vi "Launcher.vi"(8 "Quicklaunch (2)":bool, 9 "Launch Button (3)":bool, 10 "Launch Motors On (1)":bool) -> ()   [LabVIEW 2012]
uses:
  <vilib>/Rock Robotics/WPI/Solenoid/WPI_SolenoidValue.ctl
  <vilib>/Rock Robotics/WPI/Relay/WPI_RelayValue.ctl
  <vilib>/Rock Robotics/WPI/Solenoid/WPI_SolenoidSetEnum.vi
panel:
  out "Launcher On?":bool
  out "Launch Reduction":dbl
  in  "On Button Clicks":dbl
  out "Charge Up tick":dbl
  in  "Quicklaunch State":T1(ring)
  in  "Fast-Slow Variable":dbl=1.0
  in  "Charge Up Time":dbl=4000.0
  in  "Time Between Launches":dbl=2500.0
  out "Time Between tick":dbl
  out "Launch Wait tick":dbl
  in  "Launch Wait Time":dbl=500.0
  out "tick 2":dbl
  in  "time extended":dbl=500.0
  out "tick":dbl
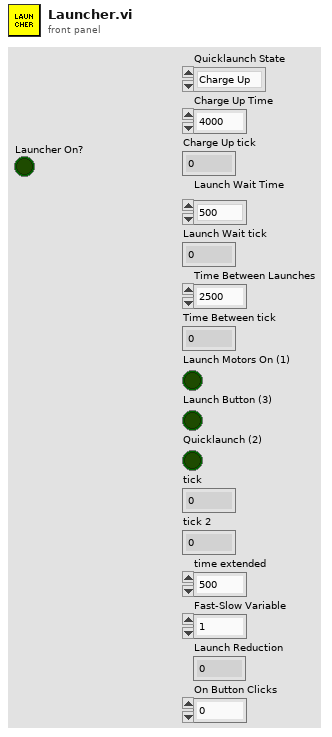
[diagram p1: front panel]
types:
  T1 = enum16{"Charge Up ", "Fire 1", "wait1", "Fire 2", "wait2", "Fire 3", "wait3", "Fire 4"}
  T2 = typedef "WPI_SolenoidValue.ctl" = enum16{"Off", "On", "Forward", "Reverse"}
  T3 = typedef "WPI_SolenoidDevRef.ctl" = cluster{"DevStatus":errorcluster, "Solenoid Module":T4, "Forward Solenoid Channel":T5, "Reverse Solenoid Channel":T5}
  T4 = typedef "FPGA_TypedefSolenoidModule.ctl" = enum16{"Solenoid Module 1", "Solenoid Module 2"}
  T5 = typedef "WPI_SolenoidChannel.ctl" = enum8{"Solenoid 1", "Solenoid 2", "Solenoid 3", "Solenoid 4", "Solenoid 5", "Solenoid 6", "Solenoid 7", "Solenoid 8", "Invalid"}
  T6 = typedef "WPI_RelayValue.ctl" = enum16{"Off", "On", "Forward", "Reverse"}
  T7 = typedef "WPI_MotorControlDeviceRef.ctl" = cluster{"DeviceStatus":errorcluster, "Type":enum16{"PWM", "CAN"}, "PWM":cluster{"Digital Module":T8, "PWM Channel":T9, "DeadBand":T10}, "CAN":cluster{"Device Number":u8, "Control Mode":T11, "Semaphore":T12, "Max Vout":dbl}, "Invert":bool, "TransformRef":T13, "InvTransformRef":T13}
  T8 = typedef "FPGA_TypedefDigitalModule.ctl" = enum16{"Digital Module 1", "Digital Module 2"}
  T9 = typedef "FPGA_DIOPWMChannel.ctl" = enum8{"PWM 1", "PWM 2", "PWM 3", "PWM 4", "PWM 5", "PWM 6", "PWM 7", "PWM 8", "PWM 9", "PWM 10", "Invalid"}
  T10 = typedef "WPI_PWMDeadband.ctl" = cluster{"Name":string, "maxPositivePwm":i32, "minPositivePwm":i32, "centerPwm":i32, "maxNegativePwm":i32, "minNegativePwm":i32, "angularRange":u16}
  T11 = typedef "WPI_CANJaguar_ControlMode.ctl" = enum8{"Percent VBus", "Current", "Speed", "Position", "Voltage"}
  T12 = typedef "Semaphore RefNum" = refnum<k1>
  T13 = typedef "WPI_PWMTransform_ConPane.ctl" = refnum<vi>
  T14 = typedef "WPI_RelayDevRef.ctl" = cluster{"DevStatus":errorcluster, "Relay Channel":T15, "Digital Module":T8, "Relay Direction":T16}
  T15 = typedef "FPGA_DIORelayChannel.ctl" = enum8{"Relay 1", "Relay 2", "Relay 3", "Relay 4", "Relay 5", "Relay 6", "Relay 7", "Relay 8", "Invalid"}
  T16 = typedef "WPI_RelayDirection.ctl" = enum16{"Both directions", "Forward only", "Reverse only"}
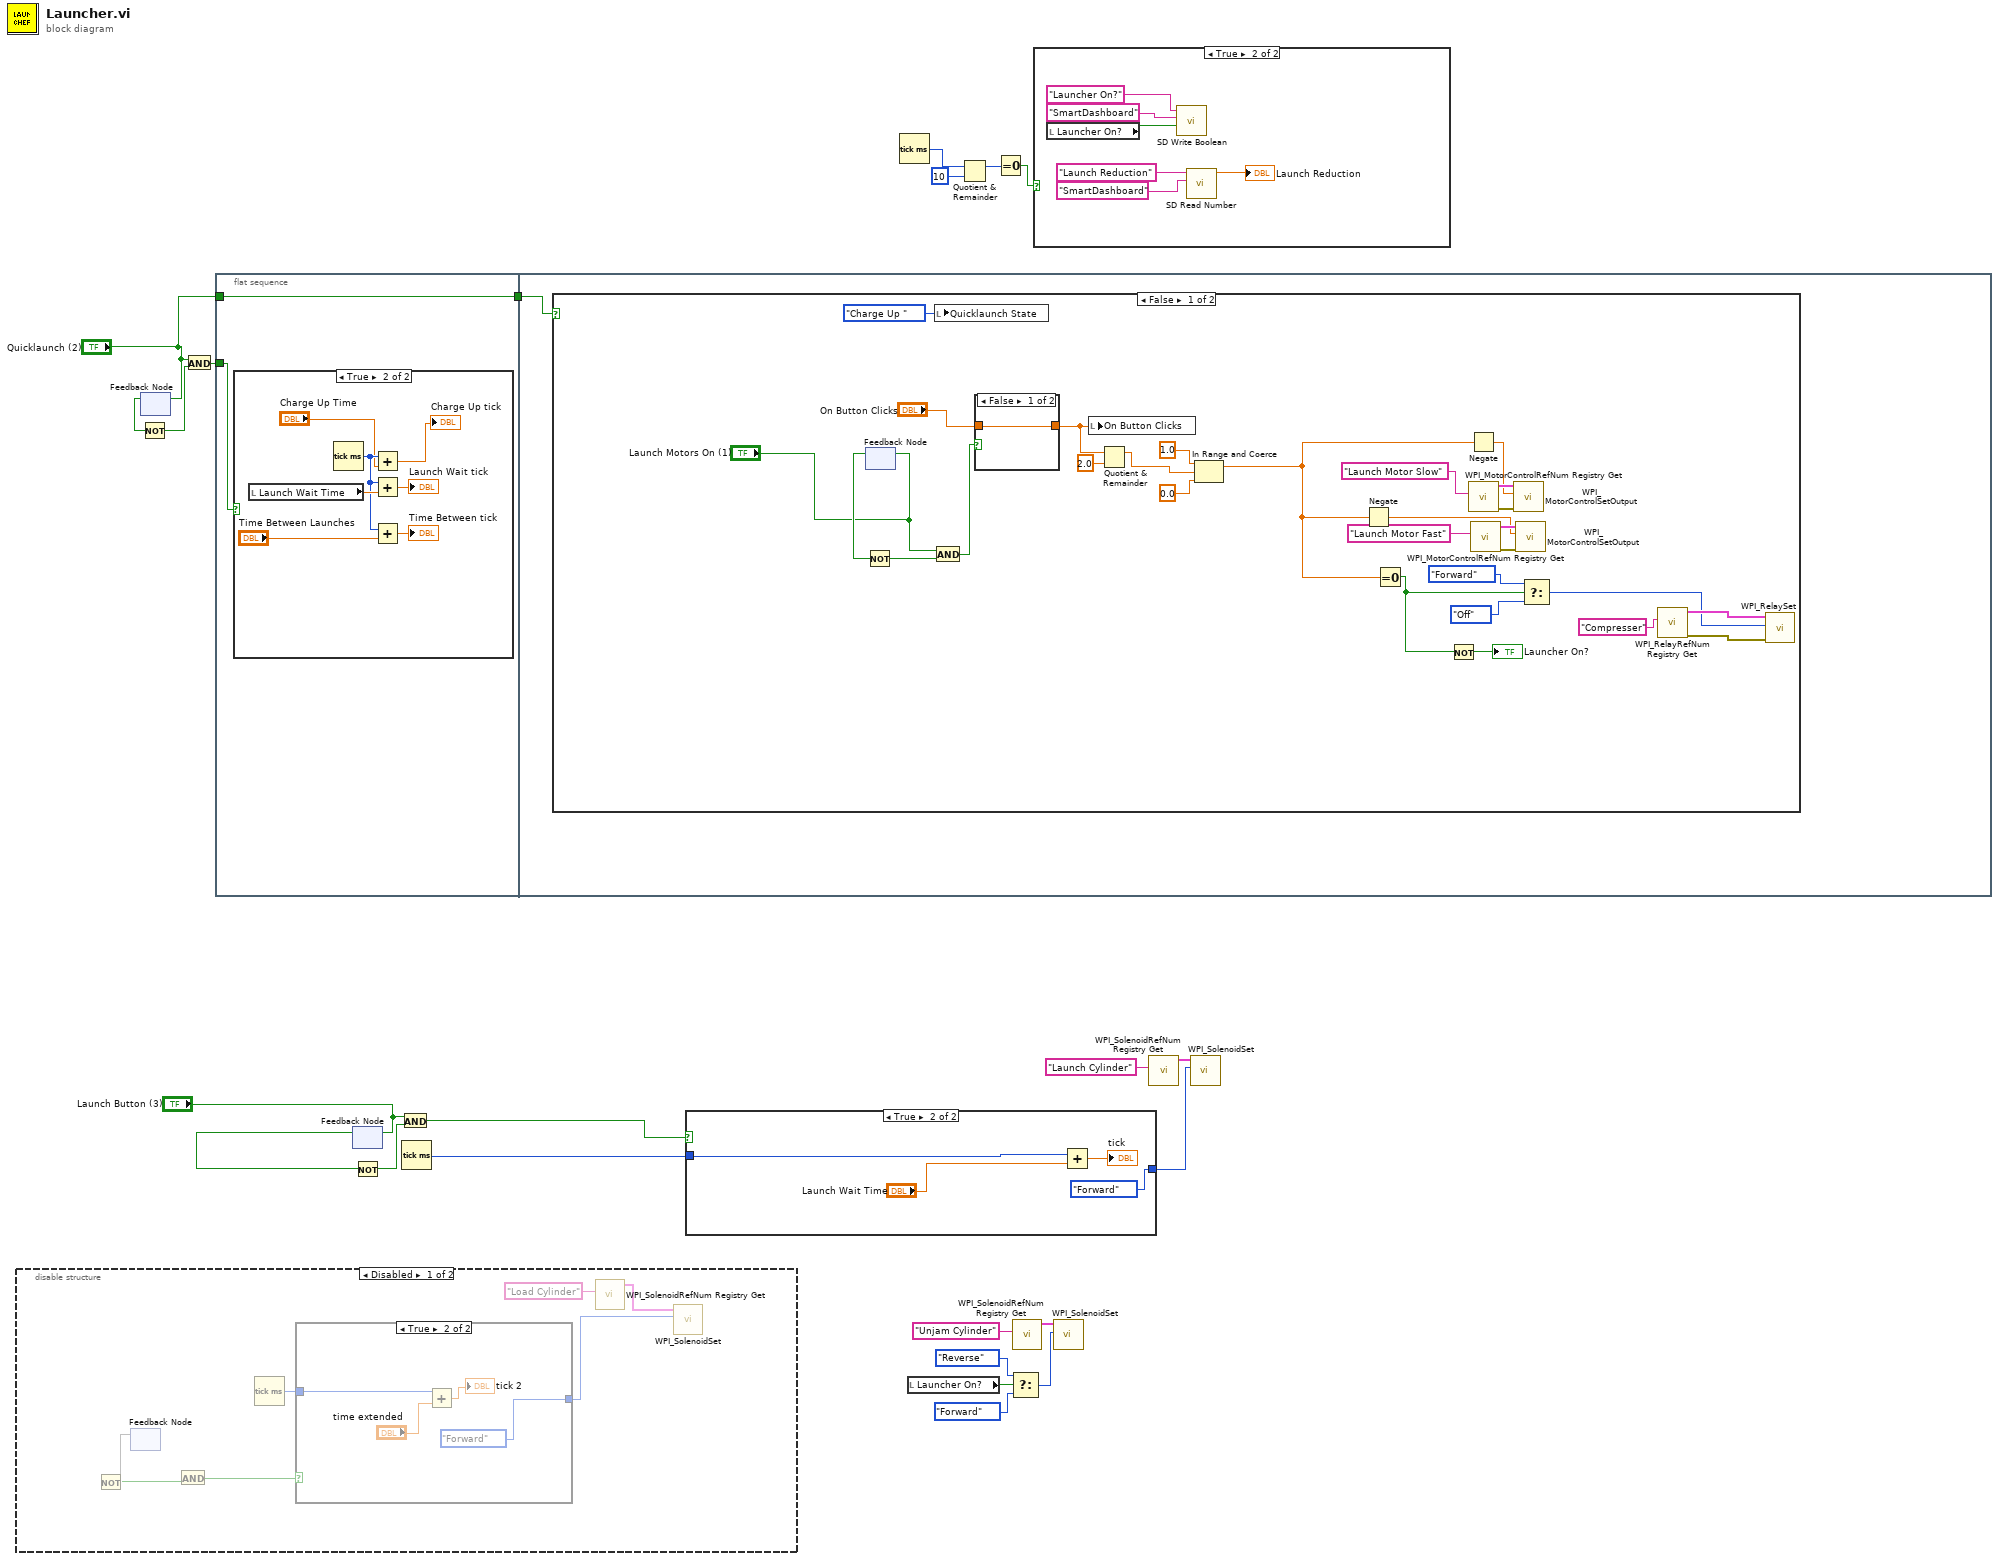
[diagram p0: block diagram]
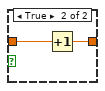
[diagram p4: hidden frame]
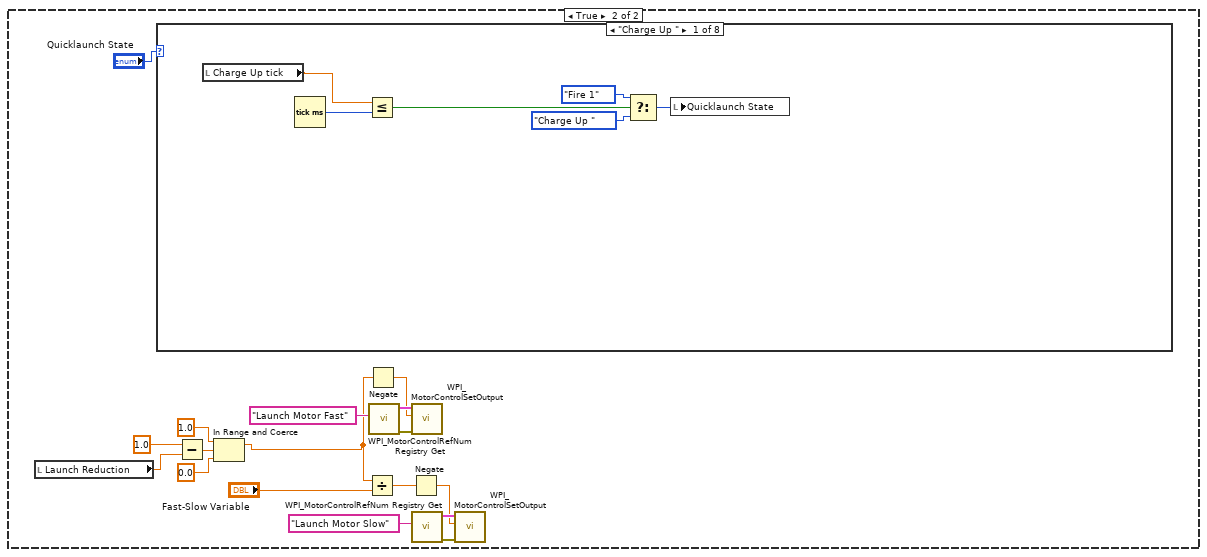
[diagram p5: hidden frame]
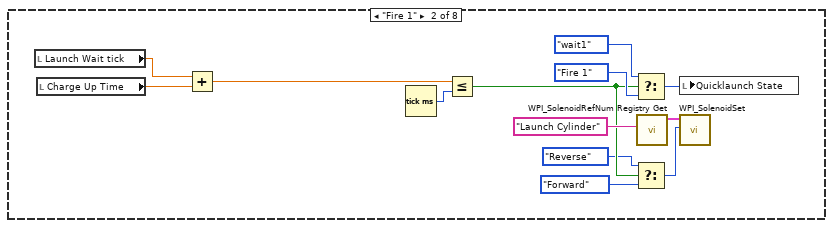
[diagram p6: hidden frame]
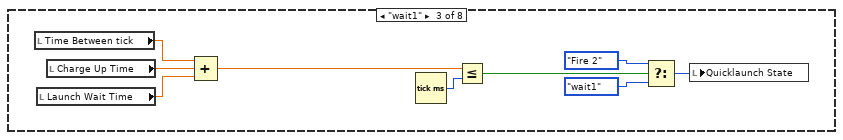
[diagram p7: hidden frame]
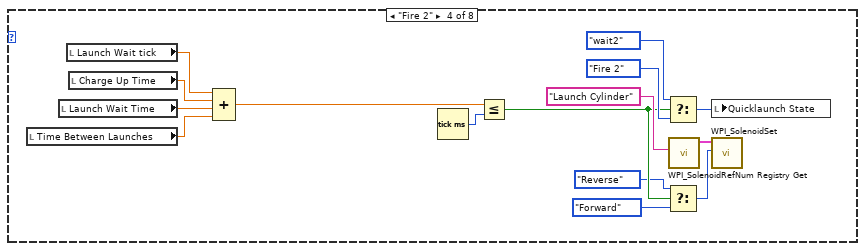
[diagram p8: hidden frame]
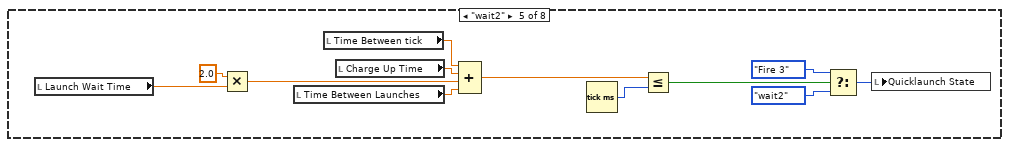
[diagram p9: hidden frame]
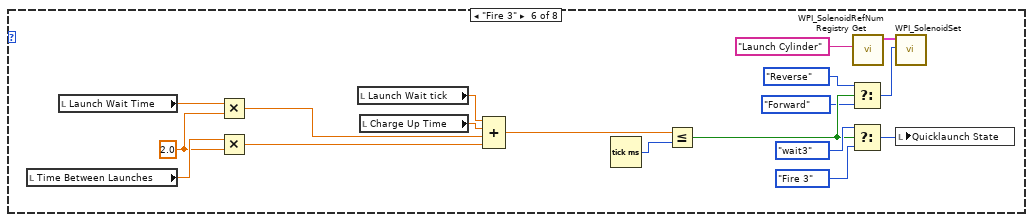
[diagram p10: hidden frame]
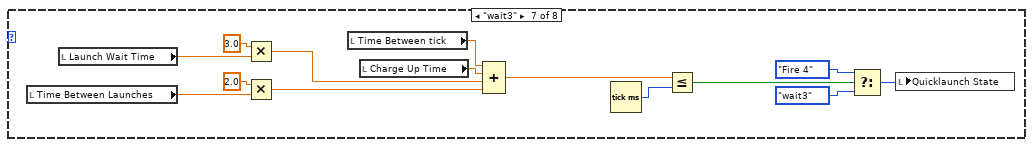
[diagram p11: hidden frame]
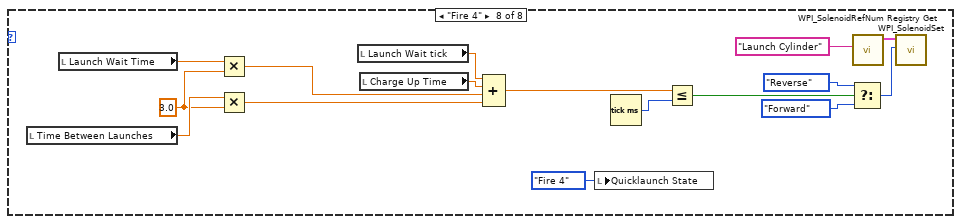
[diagram p12: hidden frame]
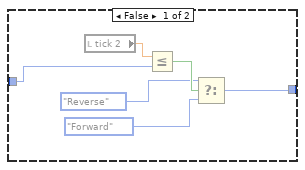
[diagram p13: hidden frame]
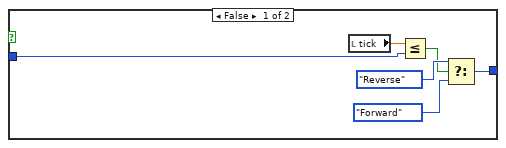
[diagram p15: hidden frame]
diagram:
  n1 = disable-structure shown="Disabled" {
    frame Disabled {
      n2 = feedback #1() -> (w30)  [unwired: 1 in]
      n3 = Not(x=w30) -> (.not. x?=w29:bool)
      n4 = feedback-in #1() -> ()  [unwired: 1 out]
      n5 = And(y=w29) -> (x .and. y?=w28:bool)  [unwired: 1 in]
      n6 = Tick Count (ms)() -> (millisecond timer value=w27:u32)
      n7 = case shown="True" w28 {
        tunnel: w27 -> [w33 w40]
        tunnel: [w36 WPI_SolenoidValue."Forward" ("Value")] -> w26
        frame False {
          n8 = local read "tick 2"() -> (w34:dbl)
          n9 = Less Or Equal?(x=w34, y=w33) -> (x <= y?=w35:bool)
          n10 = Select(t=WPI_SolenoidValue."Reverse", s=w35, f=WPI_SolenoidValue."Forward" ("Value")) -> (s? t:f=w36:T2)
        }
        frame True {
          n11 = Add(x=w40, y="time extended") -> (x+y=→"tick 2":dbl)
        }
      }
      n12 = call <vilib>:"WPI_SolenoidRefNum Registry Get.vi"("refnum name"="Load Cylinder") -> ("SolenoidDevRef"=w24:T3)  [unwired: 9 in, 1 out]
      n13 = call-poly <vilib>:"WPI_SolenoidSet.vi"("Value"=w26, "SolenoidDevRef"=w24) -> ()  [unwired: 8 in, 2 out]
    }
    frame Enabled {
    }
  }
  n14 = feedback #2() -> (w14:bool)  [unwired: 1 in]
  n15 = Not(x=w14) -> (.not. x?=w15:bool)
  n16 = feedback-in #2("Quicklaunch (2)") -> ()
  n17 = And(x="Quicklaunch (2)", y=w15) -> (x .and. y?=w13:bool)
  n18 = flat-sequence {
    tunnel: w13 -> [w42]
    tunnel: [w41] -> w12
    tunnel: "Quicklaunch (2)" -> [w41]
    tunnel: w12 -> [w50]
    frame #0 {
      n19 = case shown="True" w42 {
        frame False {
        }
        frame True {
          n20 = local read "Launch Wait Time"() -> (w49:dbl)
          n21 = Tick Count (ms)() -> (millisecond timer value=w45:u32)
          n22 = Add(x=w45, y="Charge Up Time") -> (x+y=→"Charge Up tick":dbl)
          n23 = Add(x=w45, y=w49) -> (x+y=→"Launch Wait tick":dbl)
          n24 = Add(x=w45, y="Time Between Launches") -> (x+y=→"Time Between tick":dbl)
        }
      }
    }
    frame #1 {
      n25 = case shown="False" w50 {
        frame False {
          n26 = feedback #3() -> (w67:bool)  [unwired: 1 in]
          n27 = Not(x=w67) -> (.not. x?=w61:bool)
          n28 = feedback-in #3("Launch Motors On (1)") -> ()
          n29 = And(x="Launch Motors On (1)", y=w61) -> (x .and. y?=w74:bool)
          n30 = local write "Quicklaunch State"(T1."Charge Up " ("Quicklaunch State")) -> ()
          n31 = case shown="False" w74 {
            tunnel: "On Button Clicks" -> [w79 w81]
            tunnel: [w79 w80] -> w72
            frame False {
            }
            frame True {
              n32 = Increment(x=w81) -> (x+1=w80:dbl)
            }
          }
          n33 = local write "On Button Clicks"(w72) -> ()
          n34 = Quotient & Remainder(x=w72, y=2.0) -> (x-y*floor(x/y)=w51:dbl)  [unwired: 1 out]
          n35 = In Range and Coerce(upper limit=1.0, x=w51, lower limit=0.0) -> (coerced(x)=w52:dbl)  [unwired: 1 out]
          n36 = Negate(x=w52) -> (-x=w60:dbl)
          n37 = Equal To 0?(x=w52) -> (x = 0?=w54:bool)
          n38 = Not(x=w54) -> (.not. x?=→"Launcher On?":bool)
          n39 = Negate(x=w52) -> (-x=w59:dbl)
          n40 = call <vilib>:"WPI_MotorControlRefNum Registry Get.vi"("refnum name"="Launch Motor Slow") -> ("error out"=w69:errorcluster, "MotorControlDevRef"=w68:T7)  [unwired: 9 in]
          n41 = call <vilib>:"WPI_MotorControlRefNum Registry Get.vi"("refnum name"="Launch Motor Fast") -> ("error out"=w65:errorcluster, "MotorControlDevRef"=w66:T7)  [unwired: 9 in]
          n42 = call <vilib>:"WPI_MotorControlSetOutput.vi"("error in (no error)"=w69, "Output"=w59, "MotorControlDevRef"=w68) -> ()  [unwired: 6 in, 3 out]
          n43 = call <vilib>:"WPI_MotorControlSetOutput.vi"("error in (no error)"=w65, "Output"=w60, "MotorControlDevRef"=w66) -> ()  [unwired: 6 in, 3 out]
          n44 = Select(t=WPI_RelayValue."Forward" ("RelayValue"), s=w54, f=WPI_RelayValue."Off" ("RelayValue")) -> (s? t:f=w58:T6)
          n45 = call <vilib>:"WPI_RelayRefNum Registry Get.vi"("refnum name"="Compresser") -> ("error out"=w75:errorcluster, "RelayDevRef"=w76:T14)  [unwired: 9 in]
          n46 = call <vilib>:"WPI_RelaySet.vi"("error in (no error)"=w75, "RelayValue"=w58, "RelayDevRef"=w76) -> ()  [unwired: 7 in, 2 out]
        }
        frame True {
          n47 = local read "Launch Reduction"() -> (w82:dbl)
          n48 = case shown="\"Charge Up \"" "Quicklaunch State" {
            frame "Charge Up " {
              n49 = local read "Charge Up tick"() -> (w99:dbl)
              n50 = Tick Count (ms)() -> (millisecond timer value=w103:u32)
              n51 = Less Or Equal?(x=w99, y=w103) -> (x <= y?=w102:bool)
              n52 = Select(t=T1."Fire 1", s=w102, f=T1."Charge Up ") -> (s? t:f=w104:T1)
              n53 = local write "Quicklaunch State"(w104) -> ()
            }
            frame "Fire 1" {
              n54 = local read "Launch Wait tick"() -> (w113:dbl)
              n55 = local read "Charge Up Time"() -> (w111:dbl)
              n56 = Add(x=w113, y=w111) -> (x+y=w112:dbl)
              n57 = Tick Count (ms)() -> (millisecond timer value=w117:u32)
              n58 = Less Or Equal?(x=w112, y=w117) -> (x <= y?=w108:bool)
              n59 = Select(t=T1."wait1", s=w108, f=T1."Fire 1") -> (s? t:f=w116:T1)
              n60 = Select(t=WPI_SolenoidValue."Reverse" ("Value"), s=w108, f=WPI_SolenoidValue."Forward" ("Value")) -> (s? t:f=w105:T2)
              n61 = call <vilib>:"WPI_SolenoidRefNum Registry Get.vi"("refnum name"="Launch Cylinder") -> ("SolenoidDevRef"=w110:T3)  [unwired: 9 in, 1 out]
              n62 = local write "Quicklaunch State"(w116) -> ()
              n63 = call-poly <vilib>:"WPI_SolenoidSet.vi"("Value"=w105, "SolenoidDevRef"=w110) -> ()  [unwired: 8 in, 2 out]
            }
            frame "wait1" {
              n64 = local read "Time Between tick"() -> (w119:dbl)
              n65 = local read "Launch Wait Time"() -> (w120:dbl)
              n66 = local read "Charge Up Time"() -> (w121:dbl)
              n67 = Compound Arithmetic op=ADD(w119, w121, w120) -> (w118:dbl)
              n68 = Tick Count (ms)() -> (millisecond timer value=w123:u32)
              n69 = Less Or Equal?(x=w118, y=w123) -> (x <= y?=w122:bool)
              n70 = Select(t=T1."Fire 2", s=w122, f=T1."wait1") -> (s? t:f=w126:T1)
              n71 = local write "Quicklaunch State"(w126) -> ()
            }
            frame "Fire 2" {
              n72 = local read "Time Between Launches"() -> (w128:dbl)
              n73 = local read "Launch Wait Time"() -> (w129:dbl)
              n74 = local read "Launch Wait tick"() -> (w131:dbl)
              n75 = local read "Charge Up Time"() -> (w130:dbl)
              n76 = Compound Arithmetic op=ADD(w131, w130, w129, w128) -> (w127:dbl)
              n77 = Tick Count (ms)() -> (millisecond timer value=w141:u32)
              n78 = Less Or Equal?(x=w127, y=w141) -> (x <= y?=w135:bool)
              n79 = Select(t=T1."wait2", s=w135, f=T1."Fire 2") -> (s? t:f=w140:T1)
              n80 = Select(t=WPI_SolenoidValue."Reverse" ("Value"), s=w135, f=WPI_SolenoidValue."Forward" ("Value")) -> (s? t:f=w132:T2)
              n81 = call <vilib>:"WPI_SolenoidRefNum Registry Get.vi"("refnum name"="Launch Cylinder") -> ("SolenoidDevRef"=w137:T3)  [unwired: 9 in, 1 out]
              n82 = local write "Quicklaunch State"(w140) -> ()
              n83 = call-poly <vilib>:"WPI_SolenoidSet.vi"("Value"=w132, "SolenoidDevRef"=w137) -> ()  [unwired: 8 in, 2 out]
            }
            frame "wait2" {
              n84 = local read "Launch Wait Time"() -> (w147:dbl)
              n85 = Multiply(x=2.0, y=w147) -> (x*y=w143:dbl)
              n86 = local read "Time Between Launches"() -> (w144:dbl)
              n87 = local read "Time Between tick"() -> (w146:dbl)
              n88 = local read "Charge Up Time"() -> (w148:dbl)
              n89 = Compound Arithmetic op=ADD(w146, w148, w143, w144) -> (w145:dbl)
              n90 = Tick Count (ms)() -> (millisecond timer value=w150:u32)
              n91 = Less Or Equal?(x=w145, y=w150) -> (x <= y?=w149:bool)
              n92 = Select(t=T1."Fire 3", s=w149, f=T1."wait2") -> (s? t:f=w153:T1)
              n93 = local write "Quicklaunch State"(w153) -> ()
            }
            frame "Fire 3" {
              w154 = 2.0 ("y")
              n94 = local read "Time Between Launches"() -> (w157:dbl)
              n95 = local read "Launch Wait Time"() -> (w158:dbl)
              n96 = Multiply(x=w158, y=w154) -> (x*y=w155:dbl)
              n97 = Multiply(x=w157, y=w154) -> (x*y=w156:dbl)
              n98 = local read "Launch Wait tick"() -> (w161:dbl)
              n99 = local read "Charge Up Time"() -> (w160:dbl)
              n100 = Compound Arithmetic op=ADD(w161, w160, w155, w156) -> (w159:dbl)
              n101 = Tick Count (ms)() -> (millisecond timer value=w171:u32)
              n102 = Less Or Equal?(x=w159, y=w171) -> (x <= y?=w165:bool)
              n103 = Select(t=WPI_SolenoidValue."Reverse" ("Value"), s=w165, f=WPI_SolenoidValue."Forward" ("Value")) -> (s? t:f=w162:T2)
              n104 = Select(t=T1."wait3", s=w165, f=T1."Fire 3") -> (s? t:f=w170:T1)
              n105 = call <vilib>:"WPI_SolenoidRefNum Registry Get.vi"("refnum name"="Launch Cylinder") -> ("SolenoidDevRef"=w167:T3)  [unwired: 9 in, 1 out]
              n106 = call-poly <vilib>:"WPI_SolenoidSet.vi"("Value"=w162, "SolenoidDevRef"=w167) -> ()  [unwired: 8 in, 2 out]
              n107 = local write "Quicklaunch State"(w170) -> ()
            }
            frame "wait3" {
              n108 = local read "Time Between Launches"() -> (w176:dbl)
              n109 = local read "Launch Wait Time"() -> (w179:dbl)
              n110 = Multiply(x=3.0, y=w179) -> (x*y=w175:dbl)
              n111 = Multiply(x=2.0, y=w176) -> (x*y=w173:dbl)
              n112 = local read "Time Between tick"() -> (w178:dbl)
              n113 = local read "Charge Up Time"() -> (w180:dbl)
              n114 = Compound Arithmetic op=ADD(w178, w180, w175, w173) -> (w177:dbl)
              n115 = Tick Count (ms)() -> (millisecond timer value=w182:u32)
              n116 = Less Or Equal?(x=w177, y=w182) -> (x <= y?=w181:bool)
              n117 = Select(t=T1."Fire 4", s=w181, f=T1."wait3") -> (s? t:f=w185:T1)
              n118 = local write "Quicklaunch State"(w185) -> ()
            }
            frame "Fire 4" {
              w187 = 3.0 ("y")
              n119 = local read "Time Between Launches"() -> (w190:dbl)
              n120 = local read "Launch Wait Time"() -> (w191:dbl)
              n121 = Multiply(x=w191, y=w187) -> (x*y=w188:dbl)
              n122 = Multiply(x=w190, y=w187) -> (x*y=w189:dbl)
              n123 = local read "Launch Wait tick"() -> (w194:dbl)
              n124 = local read "Charge Up Time"() -> (w193:dbl)
              n125 = Compound Arithmetic op=ADD(w194, w193, w188, w189) -> (w192:dbl)
              n126 = local write "Quicklaunch State"(T1."Fire 4" ("Quicklaunch State")) -> ()
              n127 = Tick Count (ms)() -> (millisecond timer value=w201:u32)
              n128 = Less Or Equal?(x=w192, y=w201) -> (x <= y?=w198:bool)
              n129 = Select(t=WPI_SolenoidValue."Reverse" ("Value"), s=w198, f=WPI_SolenoidValue."Forward" ("Value")) -> (s? t:f=w195:T2)
              n130 = call <vilib>:"WPI_SolenoidRefNum Registry Get.vi"("refnum name"="Launch Cylinder") -> ("SolenoidDevRef"=w200:T3)  [unwired: 9 in, 1 out]
              n131 = call-poly <vilib>:"WPI_SolenoidSet.vi"("Value"=w195, "SolenoidDevRef"=w200) -> ()  [unwired: 8 in, 2 out]
            }
          }
          n132 = Subtract(x=1.0, y=w82) -> (x-y=w86:dbl)
          n133 = In Range and Coerce(upper limit=1.0, x=w86, lower limit=0.0) -> (coerced(x)=w83:dbl)  [unwired: 1 out]
          n134 = Divide(x=w83, y="Fast-Slow Variable") -> (x/y=w90:dbl)
          n135 = Negate(x=w83) -> (-x=w89:dbl)
          n136 = call <vilib>:"WPI_MotorControlRefNum Registry Get.vi"("refnum name"="Launch Motor Fast") -> ("error out"=w92:errorcluster, "MotorControlDevRef"=w93:T7)  [unwired: 9 in]
          n137 = Negate(x=w90) -> (-x=w88:dbl)
          n138 = call <vilib>:"WPI_MotorControlSetOutput.vi"("error in (no error)"=w92, "Output"=w89, "MotorControlDevRef"=w93) -> ()  [unwired: 6 in, 3 out]
          n139 = call <vilib>:"WPI_MotorControlRefNum Registry Get.vi"("refnum name"="Launch Motor Slow") -> ("error out"=w95:errorcluster, "MotorControlDevRef"=w94:T7)  [unwired: 9 in]
          n140 = call <vilib>:"WPI_MotorControlSetOutput.vi"("error in (no error)"=w95, "Output"=w88, "MotorControlDevRef"=w94) -> ()  [unwired: 6 in, 3 out]
        }
      }
    }
  }
  n141 = feedback #4() -> (w23:bool)  [unwired: 1 in]
  n142 = feedback-in #4("Launch Button (3)") -> ()
  n143 = Not(x=w23) -> (.not. x?=w22:bool)
  n144 = And(x="Launch Button (3)", y=w22) -> (x .and. y?=w20:bool)
  n145 = Tick Count (ms)() -> (millisecond timer value=w19:u32)
  n146 = case shown="True" w20 {
    tunnel: w19 -> [w206 w211]
    tunnel: [w202 WPI_SolenoidValue."Forward" ("Value")] -> w16
    frame False {
      n147 = local read "tick"() -> (w207:dbl)
      n148 = Less Or Equal?(x=w207, y=w206) -> (x <= y?=w203:bool)
      n149 = Select(t=WPI_SolenoidValue."Reverse" ("Value"), s=w203, f=WPI_SolenoidValue."Forward" ("Value")) -> (s? t:f=w202:T2)
    }
    frame True {
      n150 = Add(x=w211, y="Launch Wait Time") -> (x+y=→"tick":dbl)
    }
  }
  n151 = Tick Count (ms)() -> (millisecond timer value=w10:u32)
  n152 = local read "Launcher On?"() -> (w1:bool)
  n153 = Quotient & Remainder(x=w10, y=u32 10) -> (x-y*floor(x/y)=w8:u32)  [unwired: 1 out]
  n154 = Equal To 0?(x=w8) -> (x = 0?=w7:bool)
  n155 = Select(t=WPI_SolenoidValue."Reverse" ("Value"), s=w1, f=WPI_SolenoidValue."Forward" ("Value")) -> (s? t:f=w2:T2)
  n156 = call <vilib>:"WPI_SolenoidRefNum Registry Get.vi"("refnum name"="Unjam Cylinder") -> ("SolenoidDevRef"=w5:T3)  [unwired: 9 in, 1 out]
  n157 = case shown="True" w7 {
    frame False {
    }
    frame True {
      n158 = local read "Launcher On?"() -> (w217:bool)
      n159 = call <vilib>:"SD Write Boolean.vi"("Boolean"=w217, "Table Prefix"="SmartDashboard", "Name"="Launcher On?") -> ()  [unwired: 7 in, 2 out]
      n160 = call <vilib>:"SD Read Number.vi"("Table Prefix"="SmartDashboard", "Name"="Launch Reduction") -> ("Numeric"=→"Launch Reduction":dbl)  [unwired: 7 in, 2 out]
    }
  }
  n161 = call-poly <vilib>:"WPI_SolenoidSet.vi"("Value"=w2, "SolenoidDevRef"=w5) -> ()  [unwired: 8 in, 2 out]
  n162 = call <vilib>:"WPI_SolenoidRefNum Registry Get.vi"("refnum name"="Launch Cylinder") -> ("SolenoidDevRef"=w17:T3)  [unwired: 9 in, 1 out]
  n163 = call-poly <vilib>:"WPI_SolenoidSet.vi"("Value"=w16, "SolenoidDevRef"=w17) -> ()  [unwired: 8 in, 2 out]
